vi "Drive_8CANSwerve.vi"(0 "FrontRightDrive":dbl, 1 "FrontRightRotation":dbl, 2 "FrontLeftDrive":dbl, 3 "FrontLeftRotation":dbl, 5 "RearLeftRotation":dbl, 7 "RearLeftDrive":dbl, 9 "RearRightRotation":dbl, 11 "RearRightDrive":dbl, 12 "Feedback Device":T1=8 items=["None"=-1, "QuadEncoder"=0, "Analog"=2, "Tachometer"=4, "Pulse Width Encoded Position"=8, "Sensor Sum (S0 + S1)"=9, "Sensor Difference (D0 - D1)"=10, "Remote Source 0"=11, "Remote Source 1"=12, "Software Emulated"=15], 13 "PIDInputs":T2) -> ()   [LabVIEW 2017]
uses:
  <vilib>/Rock Robotics/WPI/ThirdParty/Phoenix-LabVIEW/Motor Controller/Controls/CTRE_Phoenix_MotorControl_FeedbackDevice.ctl
  Users/Public/Documents/Cross The Road Electronics/Phoenix-LabVIEW/Motor Controller/Controls/CTRE_Phoenix_MotorControl_ControlMode.ctl
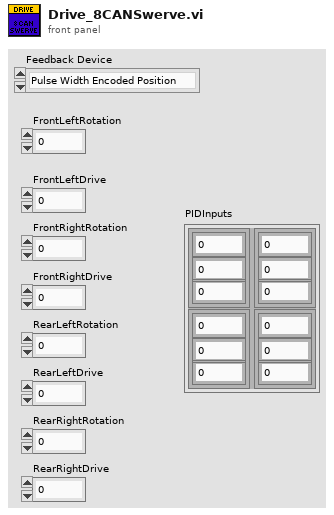
[diagram p1: front panel]
types:
  T1 = typedef "CTRE_Phoenix_MotorControl_FeedbackDevice.ctl" = i8
  T2 = cluster{"Motor1":cluster{"P":dbl, "I":dbl, "D":dbl}, "Motor3":cluster{"P":dbl, "I":dbl, "D":dbl}, "Motor2":cluster{"P":dbl, "I":dbl, "D":dbl}, "Motor4":cluster{"P":dbl, "I":dbl, "D":dbl}}
  T3 = typedef "CTRE_Phoenix_MotorControl_ControlMode.ctl" = u16
  T4 = typedef "WPI_MotorControlDeviceRef.ctl" = cluster{"DeviceStatus":errorcluster, "Type":T5, "PWM":cluster{"PWM Channel":T6, "DeadBand":T7}, "CAN":cluster{"Device Number":u8, "SetOutput VI Ref":variant, "GetOutput VI Ref":variant, "Enable VI Ref":variant, "Disable VI Ref":variant, "Data":variant}, "Invert":bool, "DIO PWM":cluster{"PWM \"Enable\" Channel":T6, "DIOChannel":T8, "PWM Rate":dbl}}
  T5 = typedef "WPI_MotorControlType.ctl" = enum16{"PWM", "CAN", "DIO PWM"}
  T6 = typedef "FPGA_DIOPWMChannel.ctl" = enum8{"PWM 0", "PWM 1", "PWM 2", "PWM 3", "PWM 4", "PWM 5", "PWM 6", "PWM 7", "PWM 8", "PWM 9", "PWM MXP 0", "PWM MXP 1", "PWM MXP 2", "PWM MXP 3", "PWM MXP 4", "PWM MXP 5", "PWM MXP 6", "PWM MXP 7", "PWM MXP 8", "PWM MXP 9", "Invalid"}
  T7 = typedef "WPI_PWMDeadband.ctl" = cluster{"Name":string, "maxPositivePwm":i32, "minPositivePwm":i32, "centerPwm":i32, "maxNegativePwm":i32, "minNegativePwm":i32, "angularRange":u16}
  T8 = typedef "FPGA_DIOChannel.ctl" = enum8{"DIO 0", "DIO 1", "DIO 2", "DIO 3", "DIO 4", "DIO 5", "DIO 6", "DIO 7", "DIO 8", "DIO 9", "DIO MXP 0", "DIO MXP 1", "DIO MXP 2", "DIO MXP 3", "DIO MXP 4", "DIO MXP 5", "DIO MXP 6", "DIO MXP 7", "DIO MXP 8", "DIO MXP 9", "DIO MXP 10", "DIO MXP 11", "DIO MXP 12", "DIO MXP 13", "DIO MXP 14", "DIO MXP 15", "SPI Port CS1", "SPI Port CS2", "SPI Port CS3", "SPI Port MISO", "SPI Port MOSI", "Invalid"}
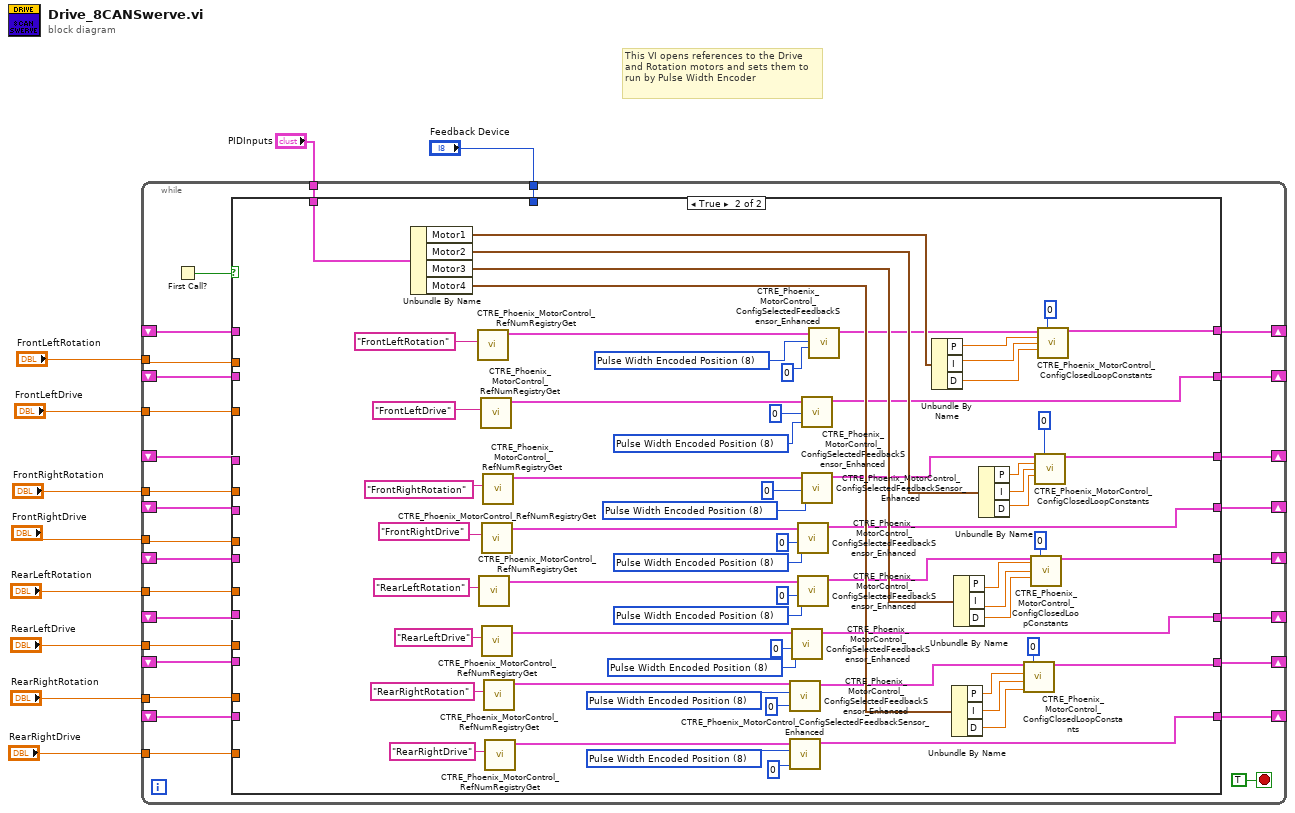
[diagram p0: block diagram]
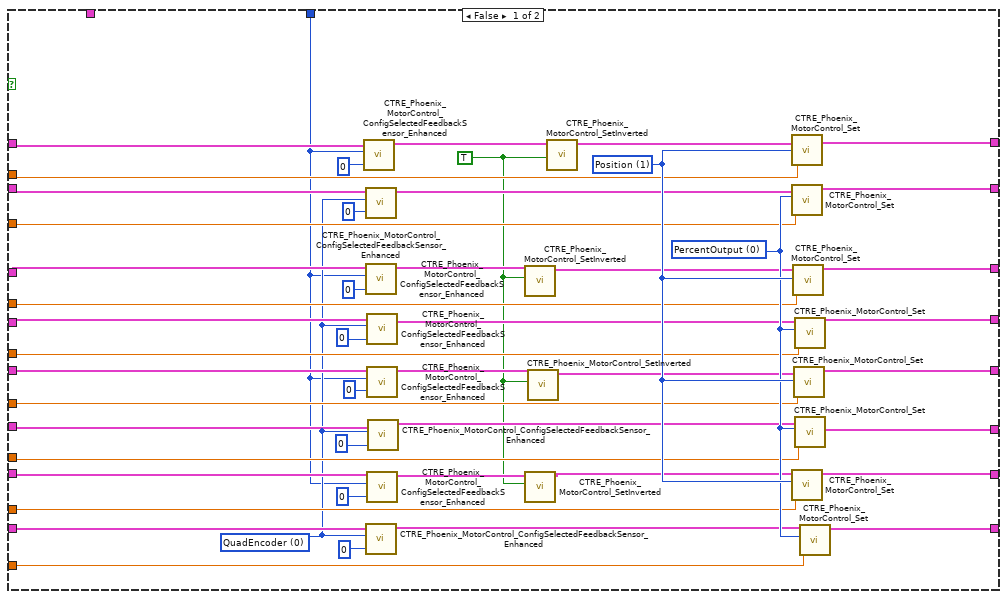
[diagram p2: hidden frame]
diagram:
  # "This VI opens references to the Drive and Rotation motors and sets them to run by Pulse Width Encoder"
  n1 = while {
    shift-right: [w38] -> _
    shift-left: _ -> [w37]
    shift-right: [w36] -> _
    shift-left: _ -> [w29]
    shift-right: [w35] -> _
    shift-left: _ -> [w28]
    shift-right: [w34] -> _
    shift-left: _ -> [w27]
    shift-right: [w33] -> _
    shift-left: _ -> [w26]
    shift-right: [w32] -> _
    shift-left: _ -> [w25]
    shift-right: [w31] -> _
    shift-left: _ -> [w24]
    shift-right: [w30] -> _
    shift-left: _ -> [w23]
    tunnel: "FrontLeftRotation" -> [w20]
    tunnel: "FrontLeftDrive" -> [w19]
    tunnel: "FrontRightRotation" -> [w18]
    tunnel: "FrontRightDrive" -> [w17]
    tunnel: "RearLeftRotation" -> [w16]
    tunnel: "RearLeftDrive" -> [w15]
    tunnel: "RearRightRotation" -> [w14]
    tunnel: "RearRightDrive" -> [w13]
    tunnel: "PIDInputs" -> [w12]
    tunnel: "Feedback Device" -> [w11]
    stop <- TRUE stop-if-true
    n2 = First Call?() -> (First Call?: T/F=w21:bool)
    n3 = case shown="True" w21 {
      tunnel: [w77 w89] -> w38
      tunnel: w37 -> [w59 _]
      tunnel: [w76 w99] -> w36
      tunnel: [w75 w90] -> w35
      tunnel: [w74 w97] -> w34
      tunnel: [w73 w91] -> w33
      tunnel: [w72 w95] -> w32
      tunnel: [w71 w92] -> w31
      tunnel: [w70 w93] -> w30
      tunnel: w29 -> [w60 _]
      tunnel: w28 -> [w61 _]
      tunnel: w27 -> [w58 _]
      tunnel: w26 -> [w57 _]
      tunnel: w25 -> [w56 _]
      tunnel: w24 -> [w55 _]
      tunnel: w23 -> [w54 _]
      tunnel: w20 -> [w85 _]
      tunnel: w19 -> [w84 _]
      tunnel: w18 -> [w83 _]
      tunnel: w17 -> [w82 _]
      tunnel: w16 -> [w81 _]
      tunnel: w15 -> [w80 _]
      tunnel: w14 -> [w79 _]
      tunnel: w13 -> [w78 _]
      tunnel: w12 -> [_ w144]
      tunnel: w11 -> [w48 _]
      frame False {
        w42 = TRUE
        w49 = T1 0 items=["None"=-1, "QuadEncoder"=0, "Analog"=2, "Tachometer"=4, "Pulse Width Encoded Position"=8, "Sensor Sum (S0 + S1)"=9, "Sensor Difference (D0 - D1)"=10, "Remote Source 0"=11, "Remote Source 1"=12, "Software Emulated"=15] ("Feedback Device")
        w86 = T3 0 items=["PercentOutput"=0, "Position"=1, "Velocity"=2, "Current"=3, "Follower"=5, "MotionProfile"=6, "MotionMagic"=7, "MotionMagicArc"=8, "MotionProfileArc"=10, "Disabled"=15] ("Control Mode")
        w87 = T3 1 items=["PercentOutput"=0, "Position"=1, "Velocity"=2, "Current"=3, "Follower"=5, "MotionProfile"=6, "MotionMagic"=7, "MotionMagicArc"=8, "MotionProfileArc"=10, "Disabled"=15] ("Control Mode")
        n4 = call <vilib>:"CTRE_Phoenix_MotorControl_ConfigSelectedFeedbackSensor_Enhanced.vi"("pidLoopIdx"=0, "Feedback Device"=w48, "PhoenixMotorControlDevRef"=w59) -> ("PhoenixMotorControlDevRef"=w44:T4)  [unwired: 7 in, 1 out]
        n5 = call <vilib>:"CTRE_Phoenix_MotorControl_ConfigSelectedFeedbackSensor_Enhanced.vi"("pidLoopIdx"=0, "Feedback Device"=w49, "PhoenixMotorControlDevRef"=w60) -> ("PhoenixMotorControlDevRef"=w50:T4)  [unwired: 7 in, 1 out]
        n6 = call <vilib>:"CTRE_Phoenix_MotorControl_ConfigSelectedFeedbackSensor_Enhanced.vi"("pidLoopIdx"=0, "Feedback Device"=w48, "PhoenixMotorControlDevRef"=w61) -> ("PhoenixMotorControlDevRef"=w45:T4)  [unwired: 7 in, 1 out]
        n7 = call <vilib>:"CTRE_Phoenix_MotorControl_ConfigSelectedFeedbackSensor_Enhanced.vi"("pidLoopIdx"=0, "Feedback Device"=w49, "PhoenixMotorControlDevRef"=w54) -> ("PhoenixMotorControlDevRef"=w53:T4)  [unwired: 7 in, 1 out]
        n8 = call <vilib>:"CTRE_Phoenix_MotorControl_ConfigSelectedFeedbackSensor_Enhanced.vi"("pidLoopIdx"=0, "Feedback Device"=w49, "PhoenixMotorControlDevRef"=w58) -> ("PhoenixMotorControlDevRef"=w51:T4)  [unwired: 7 in, 1 out]
        n9 = call <vilib>:"CTRE_Phoenix_MotorControl_ConfigSelectedFeedbackSensor_Enhanced.vi"("pidLoopIdx"=0, "Feedback Device"=w48, "PhoenixMotorControlDevRef"=w57) -> ("PhoenixMotorControlDevRef"=w46:T4)  [unwired: 7 in, 1 out]
        n10 = call <vilib>:"CTRE_Phoenix_MotorControl_ConfigSelectedFeedbackSensor_Enhanced.vi"("pidLoopIdx"=0, "Feedback Device"=w48, "PhoenixMotorControlDevRef"=w55) -> ("PhoenixMotorControlDevRef"=w47:T4)  [unwired: 7 in, 1 out]
        n11 = call <vilib>:"CTRE_Phoenix_MotorControl_ConfigSelectedFeedbackSensor_Enhanced.vi"("pidLoopIdx"=0, "Feedback Device"=w49, "PhoenixMotorControlDevRef"=w56) -> ("PhoenixMotorControlDevRef"=w52:T4)  [unwired: 7 in, 1 out]
        n12 = call <vilib>:"CTRE_Phoenix_MotorControl_SetInverted.vi"("Invert?"=w42, "PhoenixMotorControlDevRef"=w45) -> ("PhoenixMotorControlDevRef"=w39:T4)  [unwired: 8 in, 1 out]
        n13 = call <vilib>:"CTRE_Phoenix_MotorControl_SetInverted.vi"("Invert?"=w42, "PhoenixMotorControlDevRef"=w47) -> ("PhoenixMotorControlDevRef"=w41:T4)  [unwired: 8 in, 1 out]
        n14 = call <vilib>:"CTRE_Phoenix_MotorControl_SetInverted.vi"("Invert?"=w42, "PhoenixMotorControlDevRef"=w46) -> ("PhoenixMotorControlDevRef"=w40:T4)  [unwired: 8 in, 1 out]
        n15 = call <vilib>:"CTRE_Phoenix_MotorControl_SetInverted.vi"("Invert?"=w42, "PhoenixMotorControlDevRef"=w44) -> ("PhoenixMotorControlDevRef"=w43:T4)  [unwired: 8 in, 1 out]
        n16 = call <vilib>:"CTRE_Phoenix_MotorControl_Set.vi"("Output"=w85, "Control Mode"=w87, "PhoenixMotorControlDevRef"=w43) -> ("PhoenixMotorControlDevRef"=w77:T4)  [unwired: 7 in, 1 out]
        n17 = call <vilib>:"CTRE_Phoenix_MotorControl_Set.vi"("Output"=w84, "Control Mode"=w86, "PhoenixMotorControlDevRef"=w50) -> ("PhoenixMotorControlDevRef"=w76:T4)  [unwired: 7 in, 1 out]
        n18 = call <vilib>:"CTRE_Phoenix_MotorControl_Set.vi"("Output"=w79, "Control Mode"=w87, "PhoenixMotorControlDevRef"=w41) -> ("PhoenixMotorControlDevRef"=w71:T4)  [unwired: 7 in, 1 out]
        n19 = call <vilib>:"CTRE_Phoenix_MotorControl_Set.vi"("Output"=w83, "Control Mode"=w87, "PhoenixMotorControlDevRef"=w39) -> ("PhoenixMotorControlDevRef"=w75:T4)  [unwired: 7 in, 1 out]
        n20 = call <vilib>:"CTRE_Phoenix_MotorControl_Set.vi"("Output"=w81, "Control Mode"=w87, "PhoenixMotorControlDevRef"=w40) -> ("PhoenixMotorControlDevRef"=w73:T4)  [unwired: 7 in, 1 out]
        n21 = call <vilib>:"CTRE_Phoenix_MotorControl_Set.vi"("Output"=w82, "Control Mode"=w86, "PhoenixMotorControlDevRef"=w51) -> ("PhoenixMotorControlDevRef"=w74:T4)  [unwired: 7 in, 1 out]
        n22 = call <vilib>:"CTRE_Phoenix_MotorControl_Set.vi"("Output"=w80, "Control Mode"=w86, "PhoenixMotorControlDevRef"=w52) -> ("PhoenixMotorControlDevRef"=w72:T4)  [unwired: 7 in, 1 out]
        n23 = call <vilib>:"CTRE_Phoenix_MotorControl_Set.vi"("Output"=w78, "Control Mode"=w86, "PhoenixMotorControlDevRef"=w53) -> ("PhoenixMotorControlDevRef"=w70:T4)  [unwired: 7 in, 1 out]
      }
      frame True {
        w109 = T1 8 items=["None"=-1, "QuadEncoder"=0, "Analog"=2, "Tachometer"=4, "Pulse Width Encoded Position"=8, "Sensor Sum (S0 + S1)"=9, "Sensor Difference (D0 - D1)"=10, "Remote Source 0"=11, "Remote Source 1"=12, "Software Emulated"=15] ("Feedback Device")
        w110 = T1 8 items=["None"=-1, "QuadEncoder"=0, "Analog"=2, "Tachometer"=4, "Pulse Width Encoded Position"=8, "Sensor Sum (S0 + S1)"=9, "Sensor Difference (D0 - D1)"=10, "Remote Source 0"=11, "Remote Source 1"=12, "Software Emulated"=15] ("Feedback Device")
        w111 = T1 8 items=["None"=-1, "QuadEncoder"=0, "Analog"=2, "Tachometer"=4, "Pulse Width Encoded Position"=8, "Sensor Sum (S0 + S1)"=9, "Sensor Difference (D0 - D1)"=10, "Remote Source 0"=11, "Remote Source 1"=12, "Software Emulated"=15] ("Feedback Device")
        w112 = T1 8 items=["None"=-1, "QuadEncoder"=0, "Analog"=2, "Tachometer"=4, "Pulse Width Encoded Position"=8, "Sensor Sum (S0 + S1)"=9, "Sensor Difference (D0 - D1)"=10, "Remote Source 0"=11, "Remote Source 1"=12, "Software Emulated"=15] ("Feedback Device")
        w113 = T1 8 items=["None"=-1, "QuadEncoder"=0, "Analog"=2, "Tachometer"=4, "Pulse Width Encoded Position"=8, "Sensor Sum (S0 + S1)"=9, "Sensor Difference (D0 - D1)"=10, "Remote Source 0"=11, "Remote Source 1"=12, "Software Emulated"=15] ("Feedback Device")
        w114 = T1 8 items=["None"=-1, "QuadEncoder"=0, "Analog"=2, "Tachometer"=4, "Pulse Width Encoded Position"=8, "Sensor Sum (S0 + S1)"=9, "Sensor Difference (D0 - D1)"=10, "Remote Source 0"=11, "Remote Source 1"=12, "Software Emulated"=15] ("Feedback Device")
        w115 = T1 8 items=["None"=-1, "QuadEncoder"=0, "Analog"=2, "Tachometer"=4, "Pulse Width Encoded Position"=8, "Sensor Sum (S0 + S1)"=9, "Sensor Difference (D0 - D1)"=10, "Remote Source 0"=11, "Remote Source 1"=12, "Software Emulated"=15] ("Feedback Device")
        w116 = T1 8 items=["None"=-1, "QuadEncoder"=0, "Analog"=2, "Tachometer"=4, "Pulse Width Encoded Position"=8, "Sensor Sum (S0 + S1)"=9, "Sensor Difference (D0 - D1)"=10, "Remote Source 0"=11, "Remote Source 1"=12, "Software Emulated"=15] ("Feedback Device")
        n24 = Unbundle By Name(w144) -> ("Motor1"=w143:cluster{"P":dbl, "I":dbl, "D":dbl}, "Motor2"=w140:cluster{"P":dbl, "I":dbl, "D":dbl}, "Motor3"=w136:cluster{"P":dbl, "I":dbl, "D":dbl}, "Motor4"=w132:cluster{"P":dbl, "I":dbl, "D":dbl})
        n25 = call <vilib>:"CTRE_Phoenix_MotorControl_RefNumRegistryGet.vi"("refnum name"="FrontLeftRotation") -> ("PhoenixMotorControlDevRef"=w108:T4)  [unwired: 9 in, 1 out]
        n26 = call <vilib>:"CTRE_Phoenix_MotorControl_RefNumRegistryGet.vi"("refnum name"="RearLeftRotation") -> ("PhoenixMotorControlDevRef"=w104:T4)  [unwired: 9 in, 1 out]
        n27 = call <vilib>:"CTRE_Phoenix_MotorControl_RefNumRegistryGet.vi"("refnum name"="FrontLeftDrive") -> ("PhoenixMotorControlDevRef"=w107:T4)  [unwired: 9 in, 1 out]
        n28 = call <vilib>:"CTRE_Phoenix_MotorControl_RefNumRegistryGet.vi"("refnum name"="FrontRightDrive") -> ("PhoenixMotorControlDevRef"=w105:T4)  [unwired: 9 in, 1 out]
        n29 = call <vilib>:"CTRE_Phoenix_MotorControl_RefNumRegistryGet.vi"("refnum name"="RearLeftDrive") -> ("PhoenixMotorControlDevRef"=w103:T4)  [unwired: 9 in, 1 out]
        n30 = call <vilib>:"CTRE_Phoenix_MotorControl_RefNumRegistryGet.vi"("refnum name"="FrontRightRotation") -> ("PhoenixMotorControlDevRef"=w106:T4)  [unwired: 9 in, 1 out]
        n31 = call <vilib>:"CTRE_Phoenix_MotorControl_RefNumRegistryGet.vi"("refnum name"="RearRightRotation") -> ("PhoenixMotorControlDevRef"=w102:T4)  [unwired: 9 in, 1 out]
        n32 = call <vilib>:"CTRE_Phoenix_MotorControl_RefNumRegistryGet.vi"("refnum name"="RearRightDrive") -> ("PhoenixMotorControlDevRef"=w101:T4)  [unwired: 9 in, 1 out]
        n33 = call <vilib>:"CTRE_Phoenix_MotorControl_ConfigSelectedFeedbackSensor_Enhanced.vi"("pidLoopIdx"=0, "Feedback Device"=w110, "PhoenixMotorControlDevRef"=w102) -> ("PhoenixMotorControlDevRef"=w94:T4)  [unwired: 7 in, 1 out]
        n34 = call <vilib>:"CTRE_Phoenix_MotorControl_ConfigSelectedFeedbackSensor_Enhanced.vi"("pidLoopIdx"=0, "Feedback Device"=w109, "PhoenixMotorControlDevRef"=w101) -> ("PhoenixMotorControlDevRef"=w93:T4)  [unwired: 7 in, 1 out]
        n35 = call <vilib>:"CTRE_Phoenix_MotorControl_ConfigSelectedFeedbackSensor_Enhanced.vi"("pidLoopIdx"=0, "Feedback Device"=w111, "PhoenixMotorControlDevRef"=w103) -> ("PhoenixMotorControlDevRef"=w95:T4)  [unwired: 7 in, 1 out]
        n36 = call <vilib>:"CTRE_Phoenix_MotorControl_ConfigSelectedFeedbackSensor_Enhanced.vi"("pidLoopIdx"=0, "Feedback Device"=w113, "PhoenixMotorControlDevRef"=w105) -> ("PhoenixMotorControlDevRef"=w97:T4)  [unwired: 7 in, 1 out]
        n37 = call <vilib>:"CTRE_Phoenix_MotorControl_ConfigSelectedFeedbackSensor_Enhanced.vi"("pidLoopIdx"=0, "Feedback Device"=w112, "PhoenixMotorControlDevRef"=w104) -> ("PhoenixMotorControlDevRef"=w96:T4)  [unwired: 7 in, 1 out]
        n38 = call <vilib>:"CTRE_Phoenix_MotorControl_ConfigSelectedFeedbackSensor_Enhanced.vi"("pidLoopIdx"=0, "Feedback Device"=w115, "PhoenixMotorControlDevRef"=w107) -> ("PhoenixMotorControlDevRef"=w99:T4)  [unwired: 7 in, 1 out]
        n39 = call <vilib>:"CTRE_Phoenix_MotorControl_ConfigSelectedFeedbackSensor_Enhanced.vi"("pidLoopIdx"=0, "Feedback Device"=w114, "PhoenixMotorControlDevRef"=w106) -> ("PhoenixMotorControlDevRef"=w98:T4)  [unwired: 7 in, 1 out]
        n40 = call <vilib>:"CTRE_Phoenix_MotorControl_ConfigSelectedFeedbackSensor_Enhanced.vi"("pidLoopIdx"=0, "Feedback Device"=w116, "PhoenixMotorControlDevRef"=w108) -> ("PhoenixMotorControlDevRef"=w100:T4)  [unwired: 7 in, 1 out]
        n41 = Unbundle By Name(w143) -> ("P"=w88:dbl, "I"=w142:dbl, "D"=w141:dbl)
        n42 = Unbundle By Name(w132) -> ("P"=w131:dbl, "I"=w130:dbl, "D"=w129:dbl)
        n43 = Unbundle By Name(w136) -> ("P"=w135:dbl, "I"=w134:dbl, "D"=w133:dbl)
        n44 = Unbundle By Name(w140) -> ("P"=w139:dbl, "I"=w138:dbl, "D"=w137:dbl)
        n45 = call <vilib>:"CTRE_Phoenix_MotorControl_ConfigClosedLoopConstants.vi"("PhoenixMotorControlDevRef"=w94, "slotIdx"=0, "P"=w131, "I"=w130, "D"=w129) -> ("PhoenixMotorControlDevRef"=w92:T4)  [unwired: 9 in, 1 out]
        n46 = call <vilib>:"CTRE_Phoenix_MotorControl_ConfigClosedLoopConstants.vi"("PhoenixMotorControlDevRef"=w96, "slotIdx"=0, "P"=w135, "I"=w134, "D"=w133) -> ("PhoenixMotorControlDevRef"=w91:T4)  [unwired: 9 in, 1 out]
        n47 = call <vilib>:"CTRE_Phoenix_MotorControl_ConfigClosedLoopConstants.vi"("PhoenixMotorControlDevRef"=w98, "slotIdx"=0, "P"=w139, "I"=w138, "D"=w137) -> ("PhoenixMotorControlDevRef"=w90:T4)  [unwired: 9 in, 1 out]
        n48 = call <vilib>:"CTRE_Phoenix_MotorControl_ConfigClosedLoopConstants.vi"("PhoenixMotorControlDevRef"=w100, "slotIdx"=0, "P"=w88, "I"=w142, "D"=w141) -> ("PhoenixMotorControlDevRef"=w89:T4)  [unwired: 9 in, 1 out]
      }
    }
  }
